vi "Motor_Plus_Impedance_controller_monday24_G_compensation.vi"() -> ()   [LabVIEW 2016]
uses:
  <vilib>/Platform/TimedLoop/XDataNode/timing_clust.ctl
  <vilib>/Platform/TimedLoop/XDataNode/nitl_modes.ctl
  <vilib>/Platform/TimedLoop/XDataNode/wakeup.ctl
  <vilib>/Platform/TimedLoop/XDataNode/loadnilvce.vi
  <vilib>/Motion/Express/_s/nimc.ax.power.power.axis.vi
  <vilib>/Motion/Express/_s/nimc.fb.read.readExecutionData.axis.vi
  <vilib>/Motion/Express/_s/nimc.fb.straightLineMove.startStraightLineMove.axis.modeVelocity.0.vi
  <vilib>/Motion/Express/_s/nimc.fb.resetPosition.resetPosition.axis.vi
  <vilib>/Motion/Express/_s/nimc.fb.stopMove.stop.axis.modeDecelerate.vi
  <vilib>/Motion/Express/_s/nimc.ex.power.power.axis.vi
  <vilib>/platform/TimedLoop/XDataNode/XDataNode.xnode
  <vilib>/Motion/BlockNode/FB.NIMotion.xnode
  <vilib>/Platform/TimedLoop/XDataNode/XDNodeRunTimeDep.lvlib
panel:
  out "Torque 2":dbl format="%.3f"
  out "mgl value":dbl format="%#_13g"
  out "Torque 2":dbl(knob) scale=-1.0..1.0
  in  "mgl":dbl format="%#_13g"
  out "post sin":dbl format="%#_13g"
  out "pre sin":dbl format="%#_13g"
  in  "Position 2":dbl=0.25 format="%#_13g"
  out "Adjusted Motor Velocity":dbl format="%.3f"
  out "Adjusted Velocity":dbl(knob) scale=-1.0..1.0
  in  "Reset Position":bool
  in  "Position":dbl=0.25 format="%#_13g"
  in  "Speed":dbl=0.25 format="%#_12g"
  out "Torque":dbl(knob) scale=0.0..3.0
  out "Position":dbl(knob) scale=-1.0..1.0
  out "Velocity":dbl(knob) scale=-1.0..5.0
  out "Load Cell":dbl(knob) scale=0.0..10.0
  in  "Move to Position?":bool
  out "Load cell, V":dbl format="%.3f"
  out "motor torque, Nm":dbl format="%.3f"
  out "motor velocity, rev/s":dbl format="%.3f"
  out "motor position, rev":dbl format="%.3f"
  in  "STOP VI":bool
  in  "Enable Axis \nControl":bool
  in  "Enable Motor \nDrive":bool
  in  "EMERGENCY MOTOR STOP":bool
  # "Raw Data from System"
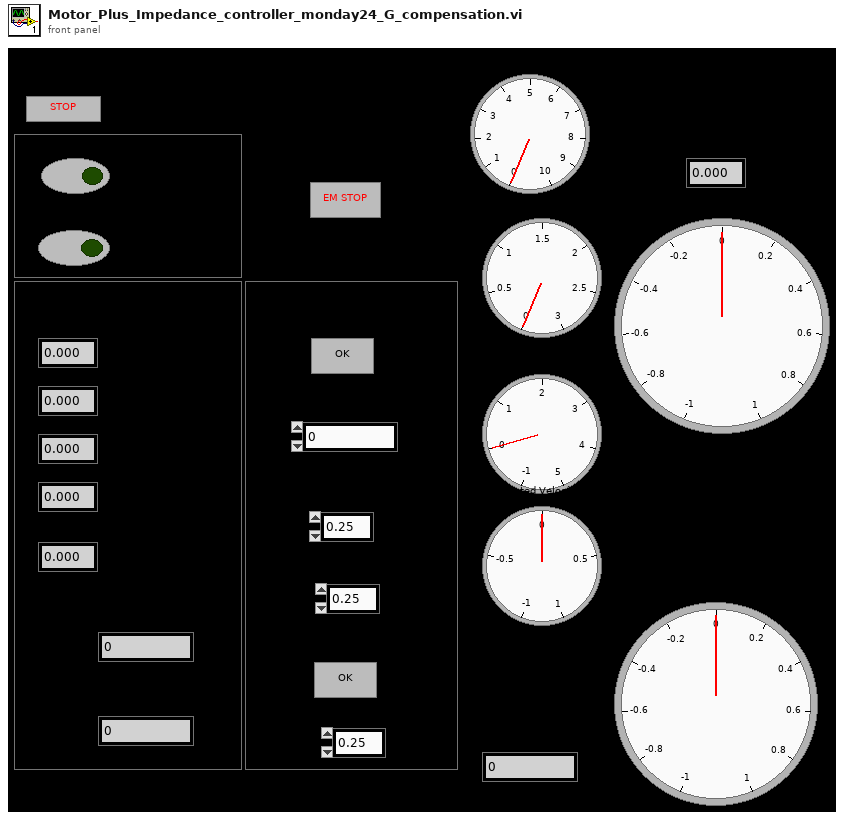
[diagram p1: front panel]
types:
  T1 = typedef "XDNodeRunTimeDep.lvlib/timing_clust.ctl" = cluster{"Expected End [f-1]":u64, "Actual End [f-1]":u64, "Finished Late? [f-1]":bool, "Expected End [i-1]":u64, "Actual End [i-1]":u64, "Finished Late? [i-1]":bool, "Expected Start [i]":u64, "Actual Start [i]":u64, "Expected Start [f]":u64, "Actual Start [f]":u64, "Source Name":string, "Structure Name":string, "Period":i64, "Deadline":i64, "Offset":i64, "Start":i64, "Priority":i32, "Timeout":i32, "Mode":T2, "Wakeup Reason":T3, "Error":errorcluster, "Source Type":string, "Secondary Source Type":string, "Global End Time":u64, "Global Start Time":u64, "Frame Duration":u64, "Iteration Duration":u64, "Assigned CPU":i32, "I/O Scan Engine Mode":u32}
  T2 = typedef "XDNodeRunTimeDep.lvlib/nitl_modes.ctl" = enum32{"No Change", "Process missed periods, maintain original phase", "Discard missed periods, maintain original phase", "Process missed periods, ignore original phase", "Discard missed periods, ignore original phase"}
  T3 = typedef "XDNodeRunTimeDep.lvlib/wakeup.ctl" = enum32{"Normal", "Aborted", "Asynchronous wakeup", "Timing source error", "Timed loop error", "Timeout"}
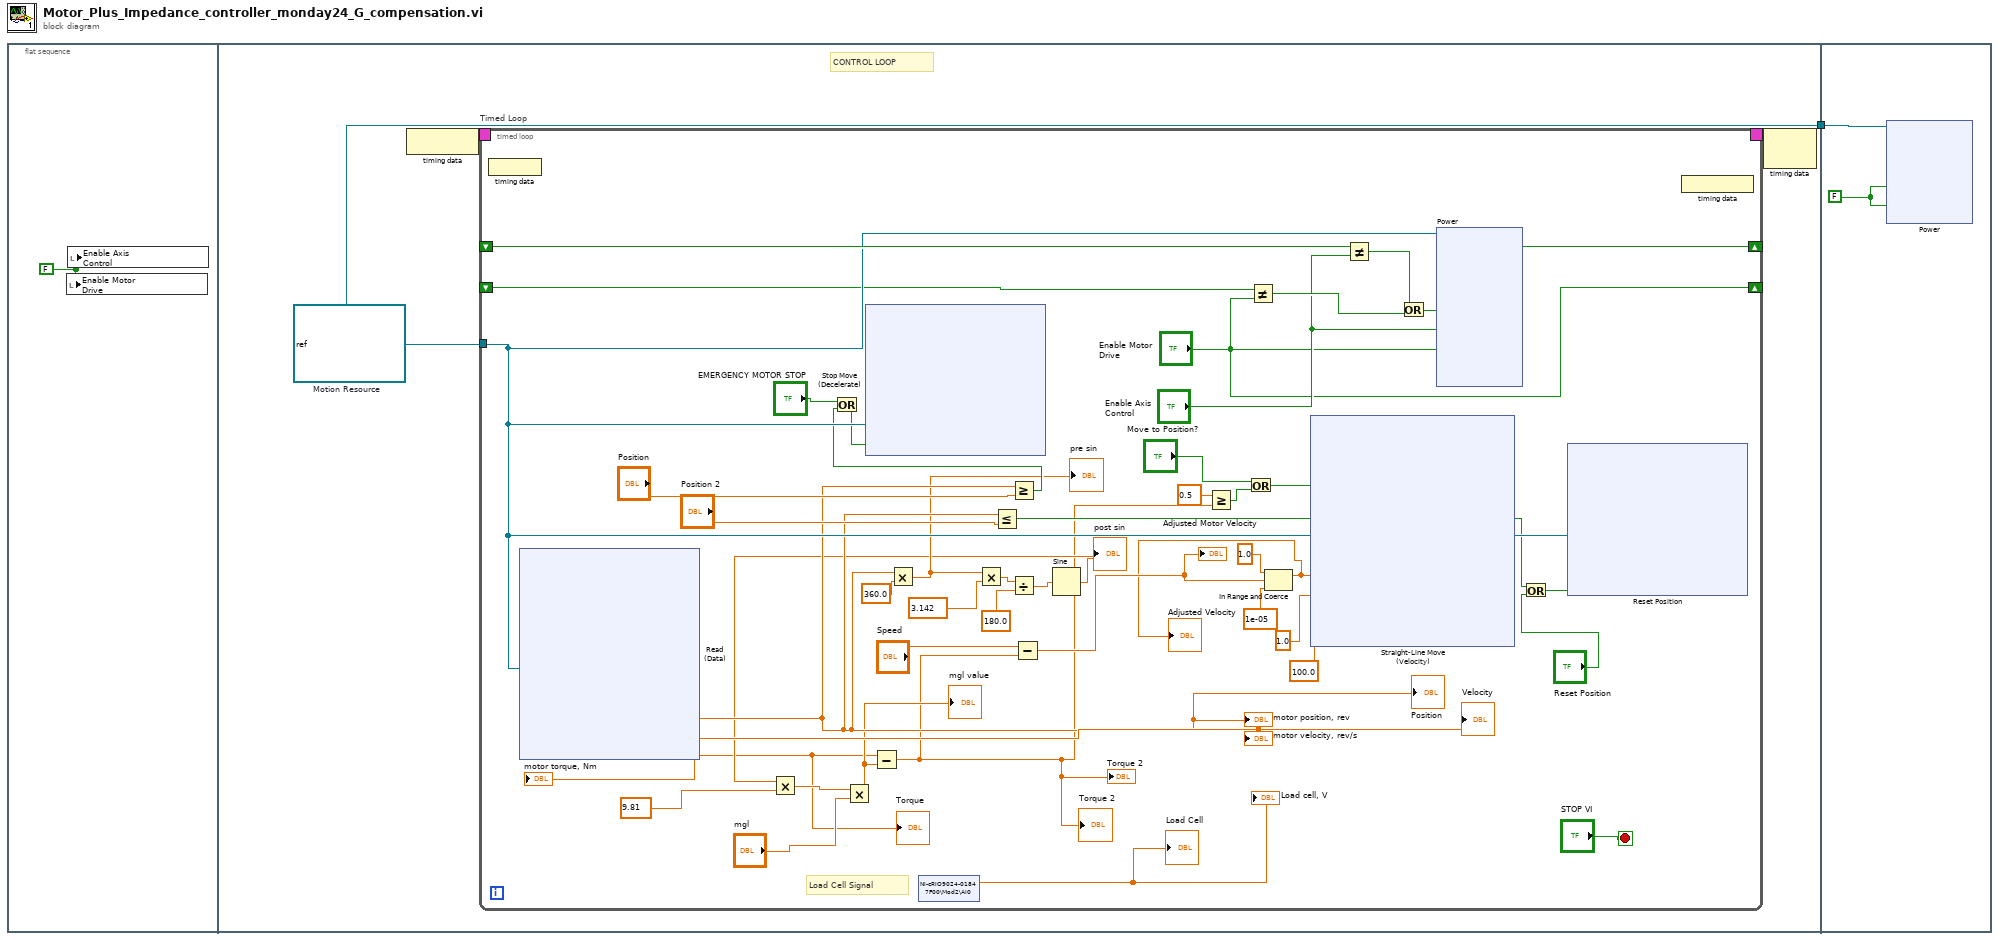
[diagram p0: block diagram]
diagram:
  n1 = flat-sequence {
    tunnel: [w5] -> w1
    tunnel: w1 -> [w128]
    frame #0 {
      w2 = FALSE
      n2 = local write "Enable Motor \nDrive"(w2) -> ()
      n3 = local write "Enable Axis \nControl"(w2) -> ()
    }
    frame #1 {
      w5 = refnum<k21> "nism://NI-cRIO9024-01847F00/Axis 1"  # Motion Resource
      # "CONTROL LOOP"
      n4 = node-c288() -> (w4:T1)
      n5 = timed-loop "Timed Loop" {
        tunnel: w5 -> [w42]
        timing: w4 -> [_]
        timing-out: [_] -> w3
        shift-right: ["Enable Axis \nControl"] -> _
        shift-left: _ -> [w49]
        shift-right: ["Enable Motor \nDrive"] -> _
        shift-left: _ -> [w30]
        stop <- "STOP VI" stop-if-true
        # "Load Cell Signal"
        n6 = node-c288() -> ()  [unwired: 1 in]
        n7 = xnode "Read\n(Data)"("resource"=w42) -> ("position"=w26:dbl, "torque"=w6:dbl, "velocity"=→"motor velocity, rev/s" →"Velocity":dbl)  [unwired: 1 in, 3 out]
        "motor position, rev" <- w26
        "motor torque, Nm" <- w6
        "Position" <- w26
        "Torque" <- w6
        n8 = Multiply(x=w26, y=360.0) -> (x*y=w21:dbl)
        "pre sin" <- w21
        n9 = shared-variable "NI-cRIO9024-01847F00\\Mod2\\AI0"() -> (→"Load cell, V" →"Load Cell":dbl)  [unwired: 1 in, 1 out]
        n10 = Multiply(x=w21, y=3.142) -> (x*y=w19:dbl)
        n11 = Less Or Equal?(x=w26, y="Position 2") -> (x <= y?=w27:bool)
        n12 = Greater Or Equal?(x=w26, y="Position") -> (x >= y?=w28:bool)
        n13 = Or(x="EMERGENCY MOTOR STOP", y=w28) -> (x .or. y?=w35:bool)
        n14 = xnode "Stop Move\n(Decelerate)"("resource"=w42, "execute"=w35) -> ()  [unwired: 1 in, 3 out]
        n15 = Divide(x=w19, y=180.0) -> (x/y=w18:dbl)
        n16 = Sine(x=w18) -> (sin(x)=w16:dbl)
        "post sin" <- w16
        n17 = Multiply(x=w16, y=9.81) -> (x*y=w23:dbl)
        n18 = Multiply(x=w23, y="mgl") -> (x*y=w8:dbl)
        "mgl value" <- w8
        n19 = Subtract(x=w6, y=w8) -> (x-y=w7:dbl)
        "Torque 2" <- w7
        "Torque 2" <- w7
        n20 = Subtract(x="Speed", y=w7) -> (x-y=w11:dbl)
        "Adjusted Motor Velocity" <- w11
        n21 = Greater Or Equal?(x=0.5, y=w7) -> (x >= y?=w15:bool)
        n22 = Or(x="Move to Position?", y=w15) -> (x .or. y?=w29:bool)
        n23 = Not Equal?(x=w30, y="Enable Motor \nDrive") -> (x != y?=w47:bool)
        n24 = In Range and Coerce(upper limit=1.0, x=w11, lower limit=1e-05) -> (coerced(x)=w9:dbl)  [unwired: 1 out]
        "Adjusted Velocity" <- w9
        n25 = xnode "Straight-Line Move\n(Velocity)"("resource"=w42, "execute"=w29, "velocity"=w9, "acceleration"=1.0, "deceleration"=100.0) -> ("resource out"=w39:refnum<k21>)  [unwired: 1 in, 2 out]
        n26 = Not Equal?(x=w49, y="Enable Axis \nControl") -> (x != y?=w48:bool)
        n27 = Or(x=w48, y=w47) -> (x .or. y?=w46:bool)
        n28 = xnode ("Power")("execute"=w46, "enable axis"="Enable Axis \nControl", "enable drive"="Enable Motor \nDrive", "resource"=w42) -> ()  [unwired: 1 in, 6 out]
        n29 = Or(x=w27, y="Reset Position") -> (x .or. y?=w38:bool)
        n30 = xnode "Reset Position"("resource"=w39, "execute"=w38) -> ()  [unwired: 2 in, 3 out]
        n31 = node-c288() -> ()  [unwired: 1 out]
      }
      n32 = node-c288(w3) -> ()  [unwired: 1 out]
    }
    frame #2 {
      w129 = FALSE
      n33 = xnode ("Power")("enable axis"=w129, "enable drive"=w129, "resource"=w128) -> ()  [unwired: 1 in, 2 out]
    }
  }
